vi "Easy XML Signature.vi"() -> ()   [LabVIEW 2016]
uses:
  <vilib>/NI/Tools/String/Tools_String.lvlib
panel:
  in  "Signature":T1
  out "Signed XML String":string
  in  "Data to Sign":T2={"Data To Secure"={"Critical Data"={"Data to protect"="Important Data", "More data to protect"="More Important Data"}}}
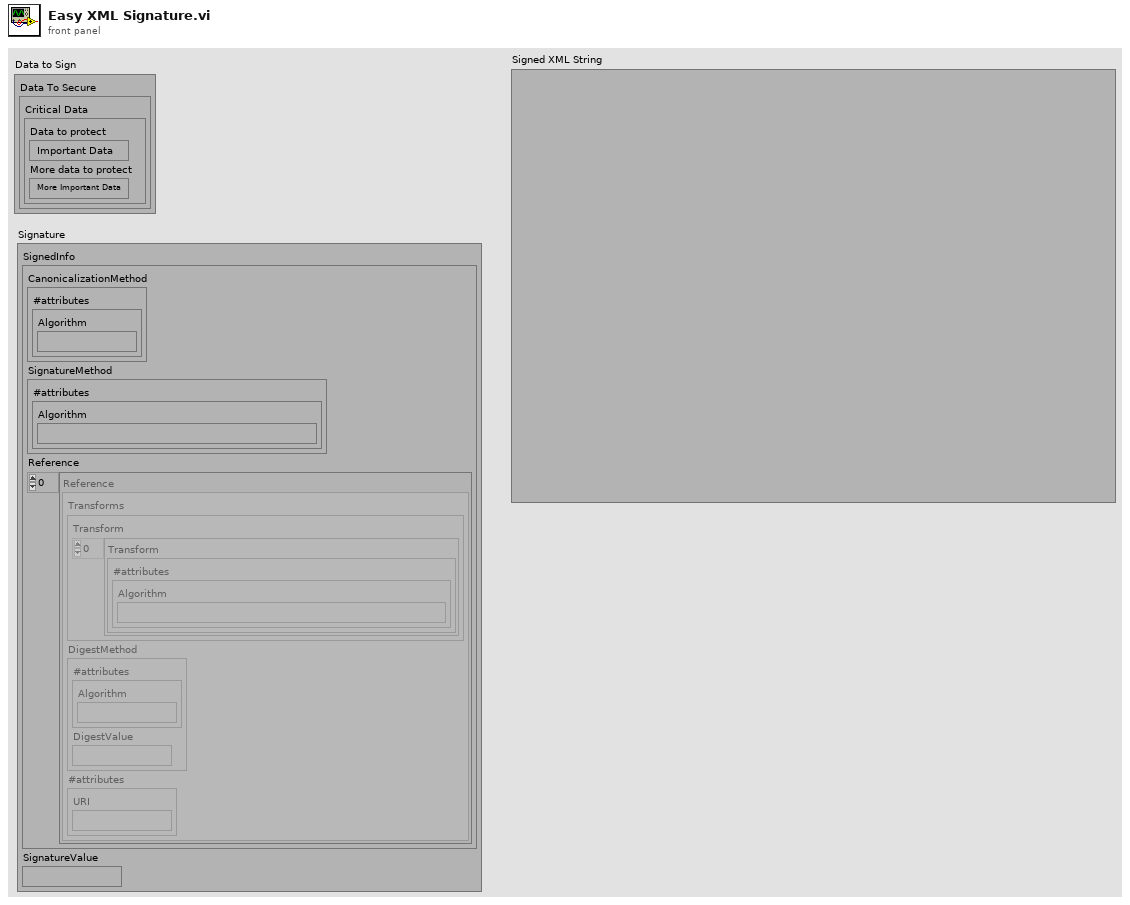
[diagram p1: front panel]
types:
  T1 = cluster{"SignedInfo":cluster{"CanonicalizationMethod":cluster{"#attributes":cluster{"Algorithm":string}}, "SignatureMethod":cluster{"#attributes":cluster{"Algorithm":string}}, "Reference":cluster{"Transforms":cluster{"Transform":cluster{"#attributes":cluster{"Algorithm":string}}[]}, "DigestMethod":cluster{"#attributes":cluster{"Algorithm":string}, "DigestValue":string}, "#attributes":cluster{"URI":string}}[]}, "SignatureValue":string}
  T2 = cluster{"Data To Secure":cluster{"Critical Data":cluster{"Data to protect":string, "More data to protect":string}}}
  T3 = enum16{"MD5", "RIPEMD160", "SHA1", "SHA256", "SHA384", "SHA512"}
  T4 = cluster{"Critical Data":cluster{"Data to protect":string, "More data to protect":string}}
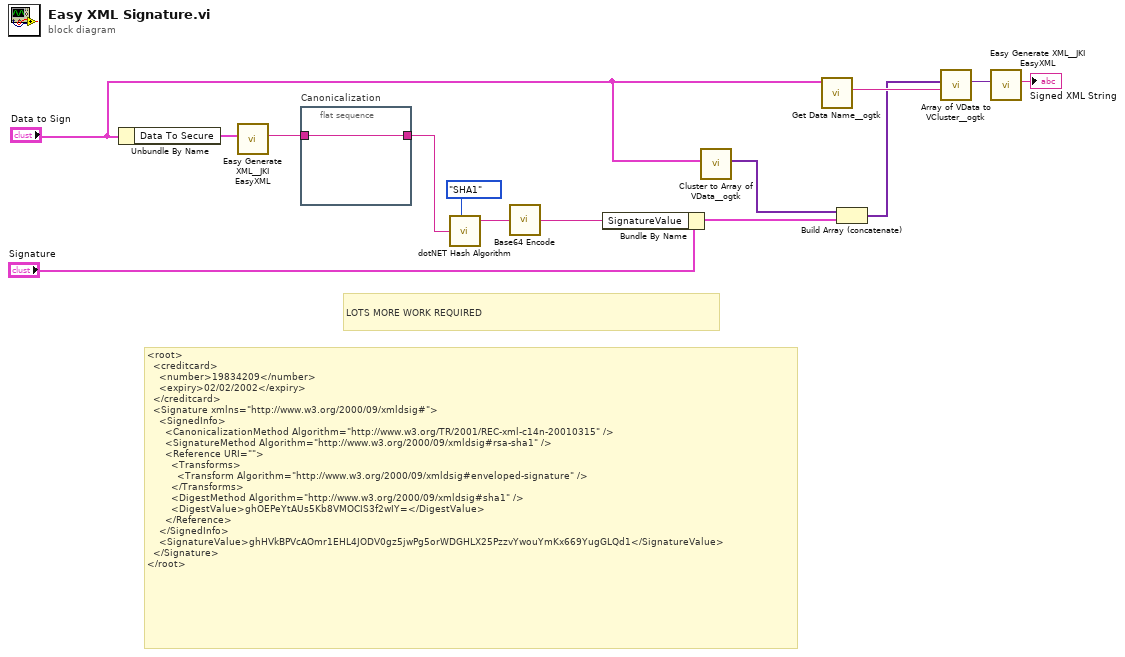
[diagram p0: block diagram]
diagram:
  # "LOTS MORE WORK REQUIRED"
  # "<root>\n  <creditcard>\n    <number>19834209</number>\n    <expiry>02/02/2002</expiry>\n  </creditcard>\n  <Signature xmlns=\"http://www.w3.org/2000/09/xmldsig#\">\n    <SignedInfo>\n      <CanonicalizationMethod Algorithm=\"http://www.w3.org/TR/2001/REC-xml-c14n-20010315\" />\n      <SignatureMethod Algorithm=\"http://www.w3.org/2000/09/xmldsig#rsa-sha1\" />\n      <Reference URI=\"\">\n        <Transforms>\n          <Transform Algorithm=\"http://www.w3.org/2000/09/xmldsig#enveloped-signature\" />\n        </Transforms>\n        <DigestMethod Algorithm=\"http://www.w3.org/2000/09/xmldsig#sha1\" />\n        <DigestValue>ghOEPeYtAUs5Kb8VMOCIS3f2wIY=</DigestValue>\n      </Reference>\n    </SignedInfo>\n    <SignatureValue>ghHVkBPVcAOmr1EHL4JODV0gz5jwPg5orWDGHLX25PzzvYwouYmKx669YugGLQd1</SignatureValue>\n  </Signature>\n</root>"
  n1 = Unbundle By Name("Data to Sign") -> ("Data To Secure"=w14:T4)
  n2 = call <vilib>:"Easy Generate XML__JKI EasyXML.vi"("LabVIEW Data"=w14) -> ("XML String"=w6:string)  [unwired: 9 in, 1 out]
  n3 = flat-sequence "Canonicalization" {
    tunnel: w6 -> [w15]
    tunnel: [w15] -> w5
    frame #0 {
    }
  }
  n4 = call "dotNET Hash Algorithm.vi"("Hash Algorithm"=T3."SHA1", "Input"=w5) -> ("Hash Base64"=w3:string)  [unwired: 3 in, 2 out]
  n5 = call <vilib>:"Base64 Encode.vi"("normal string"=w3) -> ("base64 string"=w2:string)  [unwired: 1 in]
  n6 = Bundle By Name(cluster="Signature", "SignatureValue"=w2) -> (w4:T1)
  n7 = call <userlib>:"Cluster to Array of VData__ogtk.vi"("Cluster"="Data to Sign") -> ("Array of VData"=w11:variant[])  [unwired: 9 in, 1 out]
  n8 = call <userlib>:"Get Data Name__ogtk.vi"("Data"="Data to Sign") -> ("Data Name"=w12:string)  [unwired: 8 in, 2 out]
  n9 = Build Array (concatenate)(w11, w4) -> (w9:variant[])
  n10 = call <userlib>:"Array of VData to VCluster__ogtk.vi"("Cluster Name"=w12, "Array"=w9) -> ("VCluster"=w8:variant)  [unwired: 8 in, 1 out]
  n11 = call <vilib>:"Easy Generate XML__JKI EasyXML.vi"("LabVIEW Data"=w8) -> ("XML String"=→"Signed XML String":string)  [unwired: 9 in, 1 out]
